vi "Screen_ShowProjectAbout.vi"(8 "error in":errorcluster) -> (0 "error out":errorcluster)   [LabVIEW 2014, in "hse-ui.lvlib"]
doc: "____\nHAMPEL SOFTWARE ENGINEERING v0.7.0 (2018-07-16 18:12)"
uses:
  hse-ui.lvlib
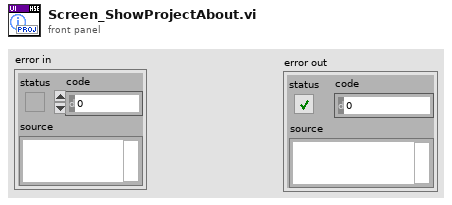
[diagram p1: front panel]
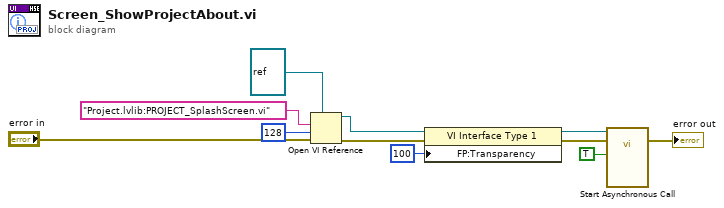
[diagram p0: block diagram]
diagram:
  n1 = Open VI Reference(type specifier VI Refnum (for type only)=refnum<vi> refnum, vi path="Project.lvlib:PROJECT_SplashScreen.vi" ("name or relative path"), options=128, error in (no error)="error in") -> (vi reference=w4:refnum<vi>, error out=w5:errorcluster)  [unwired: 2 in]
  n2 = property class="VI Interface Type 1"(reference=w4, error in=w5, "FP:Transparency"=u8 100 ("Front Panel Window:Transparency")) -> (reference out=w3:refnum<vi>, error out=w2:errorcluster)
  n3 = call-by-ref "Start Asynchronous Call"(reference=w3, error in=w2, "Allow user to close"=TRUE) -> (error out=→"error out":errorcluster)  [unwired: 11 in, 1 out]
